vi "Get Relative Timeout.vi"(1 "Timeout":T1={"mode"=enum."Relative", "deadline (ms)"=30000}) -> (0 "timeout (ms) out":i32)   [LabVIEW 2020, in "NI_Deadline.lvlib"]
uses:
  <vilib>/Utility/Deadline/NI_Deadline.lvlib
  <vilib>/Utility/Deadline/Deadline.ctl
  <vilib>/Utility/Deadline/Mode.ctl
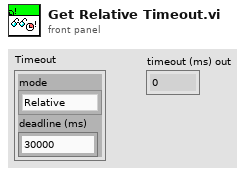
[diagram p1: front panel]
types:
  T1 = typedef "NI_Deadline.lvlib/Deadline.ctl" = cluster{"mode":T2, "deadline (ms)":u32}
  T2 = typedef "NI_Deadline.lvlib/Mode.ctl" = enum16{"Relative", "Use deadline", "Wait forever", "Nonblocking", "N/A"}
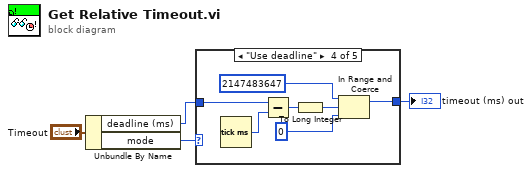
[diagram p0: block diagram]
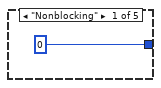
[diagram p2: hidden frame]
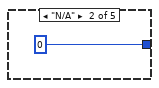
[diagram p3: hidden frame]
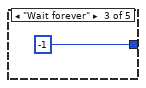
[diagram p4: hidden frame]
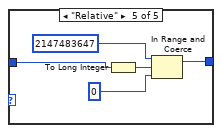
[diagram p5: hidden frame]
diagram:
  n1 = Unbundle By Name("Timeout") -> ("deadline (ms)"=w2:u32, "mode"=w3:T2)
  n2 = case shown="\"Use deadline\"" w3 {
    tunnel: [0 ("lower limit") u32 0 ("deadline (ms)") -1 ("lower limit") w9 w16] -> w1
    tunnel: w2 -> [_ _ _ w8 w15]
    frame "Nonblocking" {
    }
    frame "N/A" {
    }
    frame "Wait forever" {
    }
    frame "Use deadline" {
      n3 = Tick Count (ms)() -> (millisecond timer value=w14:u32)
      n4 = Subtract(x=w8, y=w14) -> (x-y=w11:u32)
      n5 = To Long Integer(number=w11) -> (32bit integer=w10:i32)
      n6 = In Range and Coerce(upper limit=2147483647 ("lower limit"), x=w10, lower limit=0) -> (coerced(x)=w9:i32)  [unwired: 1 out]
    }
    frame "Relative" {
      n7 = To Long Integer(number=w15) -> (32bit integer=w17:i32)
      n8 = In Range and Coerce(upper limit=2147483647 ("lower limit"), x=w17, lower limit=0) -> (coerced(x)=w16:i32)  [unwired: 1 out]
    }
  }
  "timeout (ms) out" <- w1
